vi "subConjQuat.vi"(11 "q":dbl[](array[numeric])) -> (3 "qConj":dbl[](array[numeric]))   [LabVIEW 2020]
panel:
  # "Compute the conjugate of a quaternion"
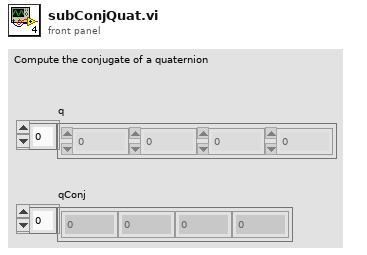
[diagram p1: front panel]
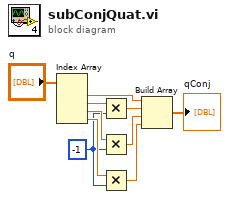
[diagram p0: block diagram]
diagram:
  w5 = -1
  n1 = Index Array(array="q") -> (element #1=w9:dbl, element #2=w8:dbl, element #3=w7:dbl, element #4=w6:dbl)  [unwired: 4 in]
  n2 = Multiply(x=w8, y=w5) -> (x*y=w4:dbl)
  n3 = Multiply(x=w7, y=w5) -> (x*y=w3:dbl)
  n4 = Multiply(x=w6, y=w5) -> (x*y=w2:dbl)
  n5 = Build Array(w9, w4, w3, w2) -> (→"qConj":dbl[])
